vi "Begin.vi"(8 "error in":errorcluster) -> (0 "error out":errorcluster)   [LabVIEW 2023]
doc: "Called before other user functions, this VI is expected to open initial I/O refnums, load in file data, and do all program initialization. Notice that the <B>error out</B> terminal is simply used for data flow. Wiring it to other structures or subVIs ensures that this VI runs first."
uses:
  Robot Global Data.vi
  <vilib>/Rock Robotics/WPI/DriverStation/WPI_DriverStationRobotMode2.ctl
  <vilib>/Rock Robotics/Network Tables/NT Write String Array.vi
  ctrl defs/ctrl pivot select.ctl
  Global INIT.vi
  ctrl defs/ctrl LIMELIGHT STREAM selector.ctl
  ctrl defs/ctrl LIMELIGHT LEDMODE selector.ctl
  ctrl defs/ctrl LIMELIGHT CAMMODE selector.ctl
  <vilib>/Rock Robotics/Network Tables/NT Write Boolean.vi
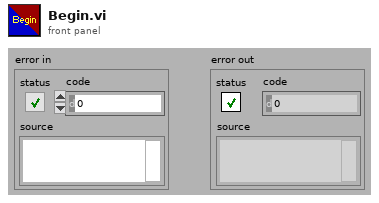
[diagram p1: front panel]
types:
  T1 = typedef "WPI_DriverStationRobotMode2.ctl" = enum16{"Autonomous Disabled", "Autonomous Enabled", "Teleop Disabled", "Teleop Enabled", "Disconnected", "Finish", "Test Disabled", "Test Enabled", "Emergency Stopped"}
  T2 = typedef "ctrl pivot select.ctl" = enum16{"geometric center", "CG", "FL", "FR", "RR", "RL", "other"}
  T3 = typedef "ctrl LIMELIGHT initialize.ctl" = cluster{"Installed?":bool, "pose":cluster{"X":dbl, "Y":dbl, "Z":dbl, "angle to horizon":dbl, "tx angle offset":dbl}}
  T4 = typedef "ctrl LIMELIGHT CAMMODE selector.ctl" = u16
  T5 = typedef "ctrl LIMELIGHT LEDMODE selector.ctl" = u16
  T6 = typedef "ctrl LIMELIGHT STREAM selector.ctl" = u16
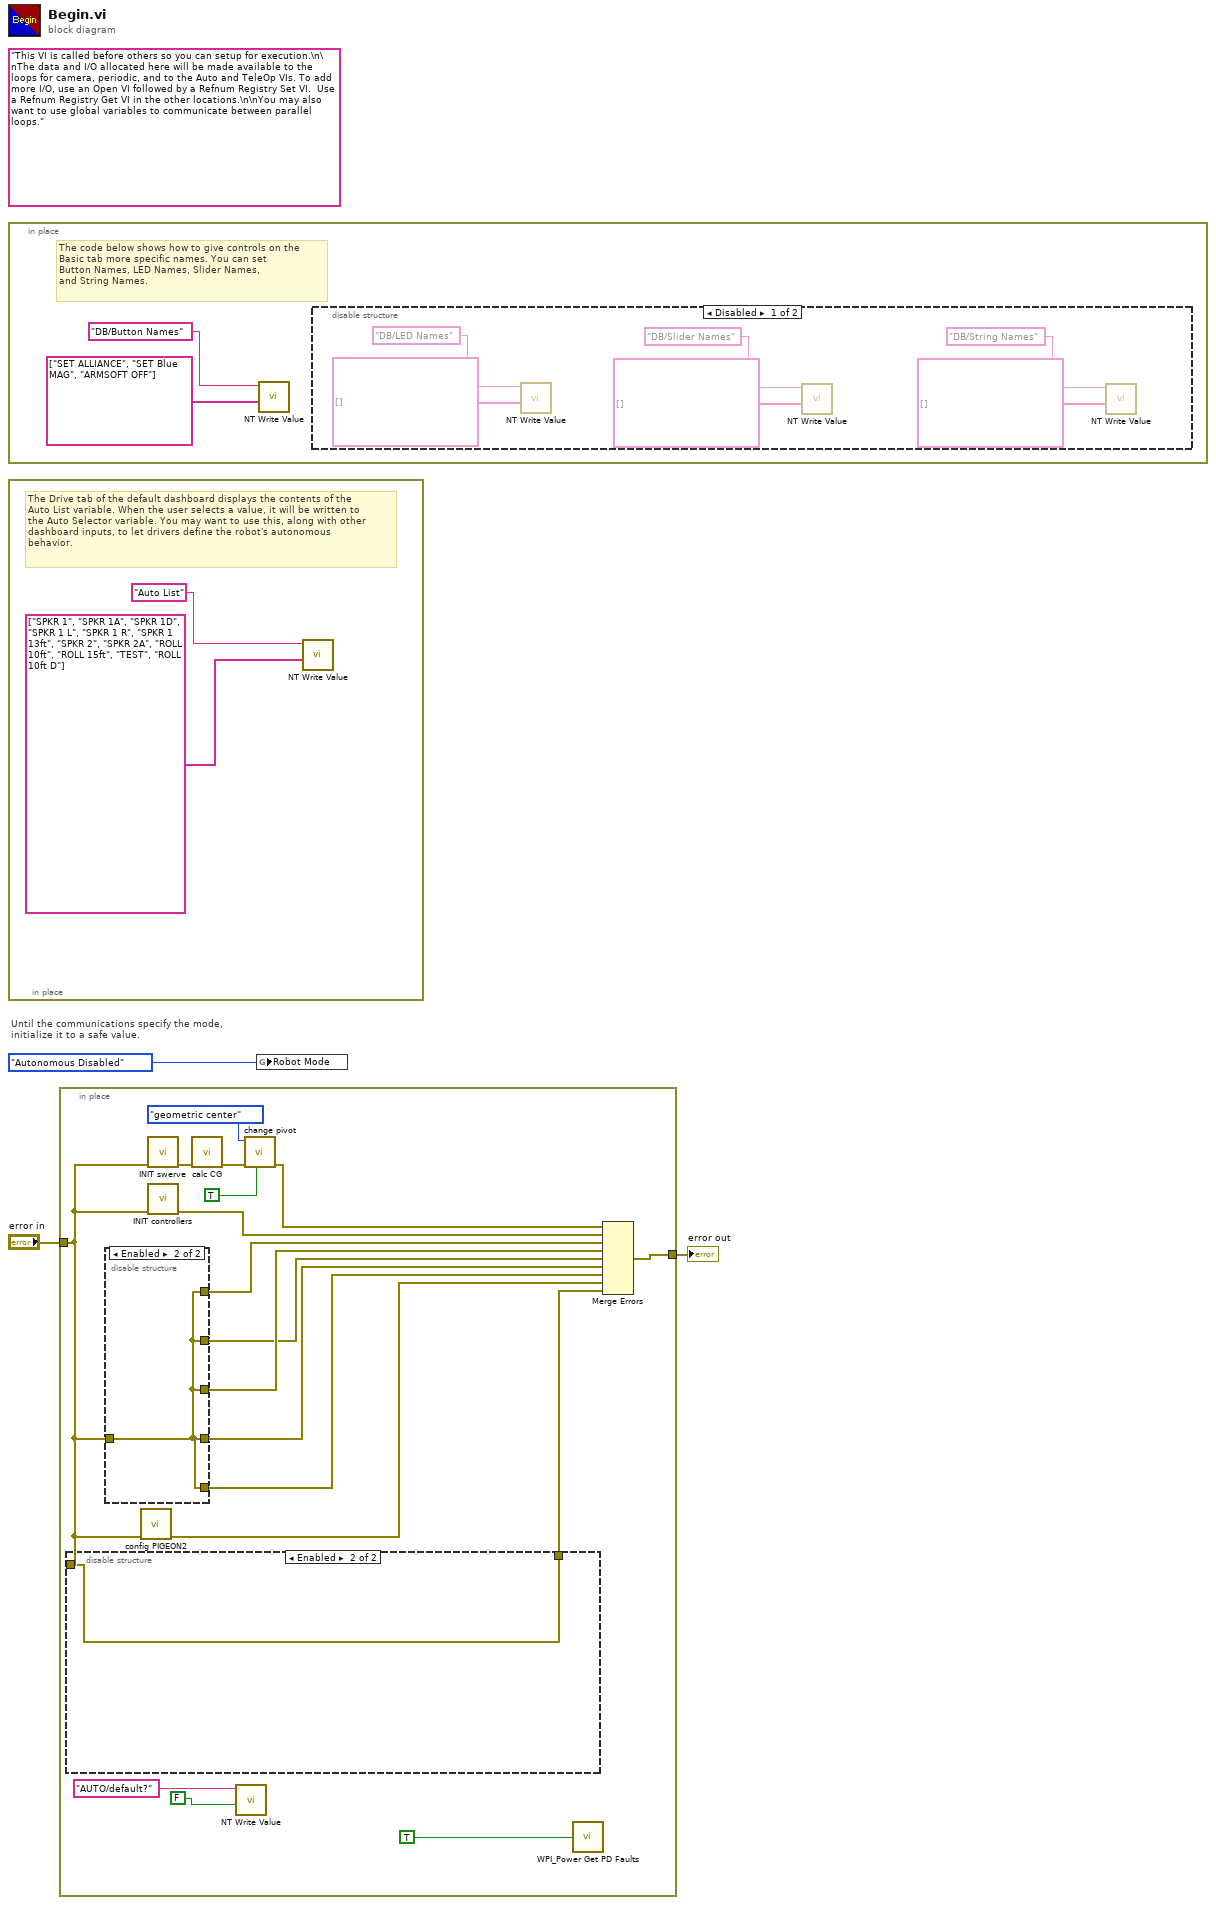
[diagram p0: block diagram]
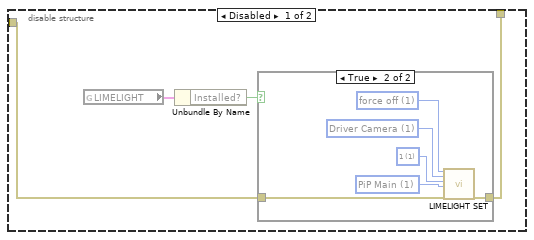
[diagram p3: hidden frame]
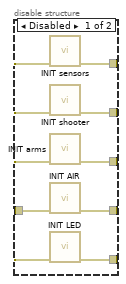
[diagram p5: hidden frame]
diagram:
  (unwired) "This VI is called before others so you can setup for execution.\n\nThe data and I/O allocated here will be made available to the loops for camera, periodic, and to the Auto and TeleOp VIs. To add more I/O, use an Open VI followed by a Refnum Registry Set VI.  Use a Refnum Registry Get VI in the other locations.\n\nYou may also want to use global variables to communicate between parallel loops."
  # "Until the communications specify the mode,\ninitialize it to a safe value."
  n1 = in-place {
    # "The code below shows how to give controls on the\nBasic tab more specific names. You can set\nButton Names, LED Names, Slider Names,\nand String Names."
    n2 = call-poly <vilib>:"NT Write Value.vi"("value"=string[] ["SET ALLIANCE", "SET Blue MAG", "ARMSOFT OFF"], "name"="DB/Button Names" ("Name")) -> ()  [unwired: 9 in, 1 out]
    n3 = disable-structure shown="Disabled" {
      frame Disabled {
        n4 = call-poly <vilib>:"NT Write Value.vi"("value"=string[] [], "name"="DB/LED Names" ("Name")) -> ()  [unwired: 9 in, 1 out]
        n5 = call-poly <vilib>:"NT Write Value.vi"("value"=string[] [], "name"="DB/Slider Names" ("Name")) -> ()  [unwired: 9 in, 1 out]
        n6 = call-poly <vilib>:"NT Write Value.vi"("value"=string[] [], "name"="DB/String Names" ("Name")) -> ()  [unwired: 9 in, 1 out]
      }
      frame Enabled {
      }
    }
  }
  n7 = in-place {
    # "The Drive tab of the default dashboard displays the contents of the\nAuto List variable. When the user selects a value, it will be written to\nthe Auto Selector variable. You may want to use this, along with other\ndashboard inputs, to let drivers define the robot's autonomous\nbehavior."
    n8 = call-poly <vilib>:"NT Write Value.vi"("value"=string[] ["SPKR 1", "SPKR 1A", "SPKR 1D", "SPKR 1 L", "SPKR 1 R", "SPKR 1 13ft", "SPKR 2", "SPKR 2A", "ROLL 10ft", "ROLL 15ft", "TEST", "ROLL 10ft D"] ("String Array"), "name"="Auto List" ("Name")) -> ()  [unwired: 9 in, 1 out]
  }
  n9 = in-place {
    in-place-border: "error in" -> [w15]
    in-place-border: [w26] -> w1
    n10 = disable-structure shown="Enabled" {
      disable-tunnel: [w33 w43] -> w16
      disable-tunnel: w15 -> [w32 w43]
      frame Disabled {
        n11 = global read "Global INIT.vi" "LIMELIGHT"() -> (w35:T3)
        n12 = Unbundle By Name(w35) -> ("Installed?"=w34:bool)
        n13 = case shown="True" w34 {
          tunnel: [w36 w42] -> w33
          tunnel: w32 -> [w36 w41]
          frame False {
          }
          frame True {
            w37 = T4 1 items=["Vision processor", "Driver Camera"] ("camMode")
            w38 = T5 1 items=["default to current pipeline", "force off", "force blink", "force on"] ("ledMode")
            w39 = T6 1 items=["standard side-by-side", "PiP Main", "PiP Secondary"] ("stream")
            w40 = u16 1 items=["0", "1", "2", "3", "4", "5", "6", "7", "8", "9"] ("pipeline")
            n14 = call "LIMELIGHT SET.vi"("ledMode"=w38, "camMode"=w37, "pipeline"=w40, "stream"=w39, "error in (no error)"=w41) -> ("error out"=w42:errorcluster)  [unwired: 14 in]
          }
        }
      }
      frame Enabled {
      }
    }
    n15 = disable-structure shown="Enabled" {
      disable-tunnel: [w49 w50] -> w25
      disable-tunnel: [w48 w50] -> w24
      disable-tunnel: [w47 w50] -> w23
      disable-tunnel: [w46 w50] -> w22
      disable-tunnel: [w45 w50] -> w21
      disable-tunnel: w15 -> [w44 w50]
      frame Disabled {
        n16 = call "INIT sensors.vi"("error in (no error)"=w44) -> ("error out"=w45:errorcluster)  [unwired: 10 in]
        n17 = call "INIT shooter.vi"("error in (no error)"=w44) -> ("error out"=w46:errorcluster)  [unwired: 10 in]
        n18 = call "INIT arms.vi"("error in (no error)"=w44) -> ("error out"=w48:errorcluster)  [unwired: 10 in]
        n19 = call "INIT AIR.vi"("error in (no error)"=w44) -> ("error out"=w47:errorcluster)  [unwired: 10 in]
        n20 = call "INIT LED.vi"("error in (no error)"=w44) -> ("error out"=w49:errorcluster)  [unwired: 10 in]
      }
      frame Enabled {
      }
    }
    n21 = call "config PIGEON2.vi"("error in (no error)"=w15) -> ("error out"=w14:errorcluster)  [unwired: 10 in]
    n22 = call "INIT swerve.vi"("error in (no error)"=w15) -> ("error out"=w31:errorcluster)  [unwired: 10 in]
    n23 = call "INIT controllers.vi"("error in (no error)"=w15) -> ("error out"=w27:errorcluster)  [unwired: 10 in]
    n24 = call "calc CG.vi"("error in (no error)"=w31) -> ("error out"=w30:errorcluster)  [unwired: 10 in]
    n25 = call-poly <vilib>:"NT Write Value.vi"("value"=FALSE, "name"="AUTO/default?") -> ()  [unwired: 9 in, 1 out]
    n26 = call "change pivot.vi"("force recalc?"=TRUE, "error in (no error)"=w30, "select pivot point"=ctrl_pivot_select."geometric center") -> ("error out"=w28:errorcluster)  [unwired: 8 in]
    n27 = call <vilib>:"WPI_Power Get PD Faults.vi"("Clear Sticky Faults"=TRUE) -> ()  [unwired: 11 in, 4 out]
    n28 = Merge Errors(w28, w27, w21, w24, w22, w23, w25, w14, w16) -> (w26:errorcluster)
  }
  "error out" <- w1
  n29 = global write "Robot Global Data.vi" "Robot Mode"(WPI_DriverStationRobotMode2."Autonomous Disabled" ("Robot Mode")) -> ()
